vi "LC Type to PGSQL Paths.vi"(8 "error in (no error)":errorcluster, 10 "LC Type":T1, 11 "FP-TC-Shared in":refnum<class "FP-TC-Shared.lvclass">) -> (0 "error out":errorcluster, 3 "FP-TC-Shared out":refnum<class "FP-TC-Shared.lvclass">)   [LabVIEW 2019, in "FP-TC-Shared.lvclass"]
uses:
  FP-TC-Shared.lvclass
  typedefs/LC Type--Enum.ctl
  FP-TC-Shared.lvclass/FP-TC-Shared.ctl
  <userlib>/LevyLab/Instrument Framework/SMOs/Configuration/Configuration.lvclass/Configuration.ctl
  <userlib>/LevyLab/Instrument Framework/SMOs/Configuration/Configuration.lvclass
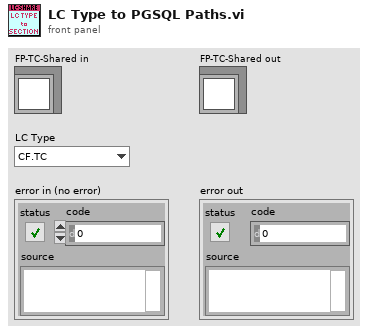
[diagram p1: front panel]
types:
  T1 = typedef "FP-TC-Shared.lvclass/LC Type--Enum.ctl" = enum16{"CF.TC", "CF.TC.Z", "CF.FP", "MNK.TC", "MNK.TC.Z", "MNK.FP"}
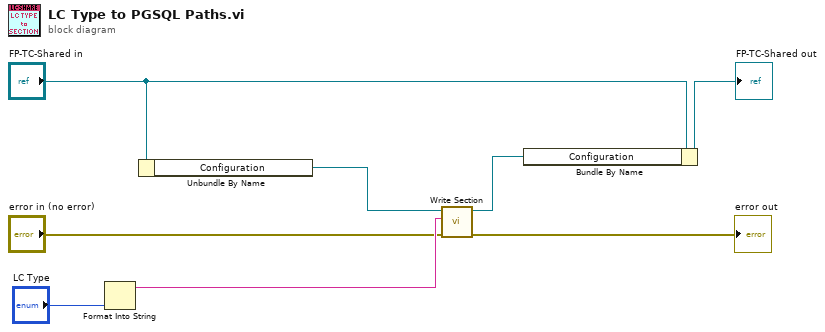
[diagram p0: block diagram]
diagram:
  n1 = Format Into String("LC Type") -> (resulting string=w4:string)  [unwired: 3 in, 1 out]
  n2 = Unbundle By Name("FP-TC-Shared in") -> ("Configuration"=w2:refnum<class "Configuration.lvclass">)
  n3 = call <userlib>:"Write Section.vi"("error in (no error)"="error in (no error)", "Section"=w4, "Configuration in"=w2) -> ("error out"=→"error out":errorcluster, "Configuration out"=w7:refnum<class "Configuration.lvclass">)  [unwired: 7 in]
  n4 = Bundle By Name(cluster="FP-TC-Shared in", "Configuration"=w7) -> (→"FP-TC-Shared out":refnum<class "FP-TC-Shared.lvclass">)
